vi "DevRef Data Base fg.vi"(0 "Menu":T12, 1 "Shooter Solenoid DevRef":T8={"DevStatus"={"status"=FALSE, "code"=0, "source"=""}, "Solenoid Module"=enum."Solenoid Module 1", "Forward Solenoid Channel"=enum."Invalid", "Reverse Solenoid Channel"=enum."Invalid"}, 2 "Latch Solenoid DevRef":T8={"DevStatus"={"status"=FALSE, "code"=0, "source"=""}, "Solenoid Module"=enum."Solenoid Module 1", "Forward Solenoid Channel"=enum."Invalid", "Reverse Solenoid Channel"=enum."Invalid"}, 3 "Right Up DevRef":T1={"DevStatus"={"status"=FALSE, "code"=0, "source"=""}, "DIO Channel"=enum."Invalid", "Digital Module"=enum."Digital Module 1"}, 4 "Right Down DevRef":T1={"DevStatus"={"status"=FALSE, "code"=0, "source"=""}, "DIO Channel"=enum."Invalid", "Digital Module"=enum."Digital Module 1"}, 5 "Hold Sensor DevRef":T1={"DevStatus"={"status"=FALSE, "code"=0, "source"=""}, "DIO Channel"=enum."Invalid", "Digital Module"=enum."Digital Module 1"}, 6 "2 Ball DevRef":T1={"DevStatus"={"status"=FALSE, "code"=0, "source"=""}, "DIO Channel"=enum."Invalid", "Digital Module"=enum."Digital Module 1"}, 7 "Arm Encoder DevRef":T4={"DevStatus"={"status"=FALSE, "code"=0, "source"=""}, "EncoderIndex"=enum."Invalid", "CounterIndex"=enum."Invalid", "DistancePerCount"=1.0, "Decoding Type"=enum."4x"}, 10 "DevRef to Get":T11) -> (20 "Selected Solenoid":T8={"DevStatus"={"status"=FALSE, "code"=0, "source"=""}, "Solenoid Module"=enum."Solenoid Module 1", "Forward Solenoid Channel"=enum."Invalid", "Reverse Solenoid Channel"=enum."Invalid"}, 21 "Selected Sensor":T1, 22 "Selected Encoder":T4={"DevStatus"={"status"=FALSE, "code"=0, "source"=""}, "EncoderIndex"=enum."Invalid", "CounterIndex"=enum."Invalid", "DistancePerCount"=1.0, "Decoding Type"=enum."4x"})   [LabVIEW 2013]
uses:
  <vilib>/Rock Robotics/WPI/Solenoid/WPI_SolenoidDevRef.ctl
  <vilib>/Rock Robotics/SystemInterfaces/Typedef/FPGA_TypedefSolenoidModule.ctl
  <vilib>/Rock Robotics/WPI/Solenoid/WPI_SolenoidChannel.ctl
  <vilib>/Rock Robotics/WPI/DigitalInput/WPI_DigitalInputDevRef.ctl
  <vilib>/Rock Robotics/SystemInterfaces/DIO/FPGA_DIOChannel.ctl
  <vilib>/Rock Robotics/SystemInterfaces/Typedef/FPGA_TypedefDigitalModule.ctl
  typedefs/fg_typedef.ctl
  typedefs/DevRef Type.ctl
  <vilib>/Rock Robotics/WPI/Encoder/WPI_EncoderDevRef.ctl
  <vilib>/Rock Robotics/SystemInterfaces/Encoder/FPGA_EncoderIdx.ctl
  <vilib>/Rock Robotics/SystemInterfaces/Counter/FPGA_CounterCtrSystemIndex.ctl
  <vilib>/Rock Robotics/WPI/Encoder/WPI_EncoderType.ctl
panel:
  # "A Functional Global that stores refnums for \ncommonly used devices \nso as to not need to get them repeatedly"
  # "it is only set once"
  # "Option to Select Also..."
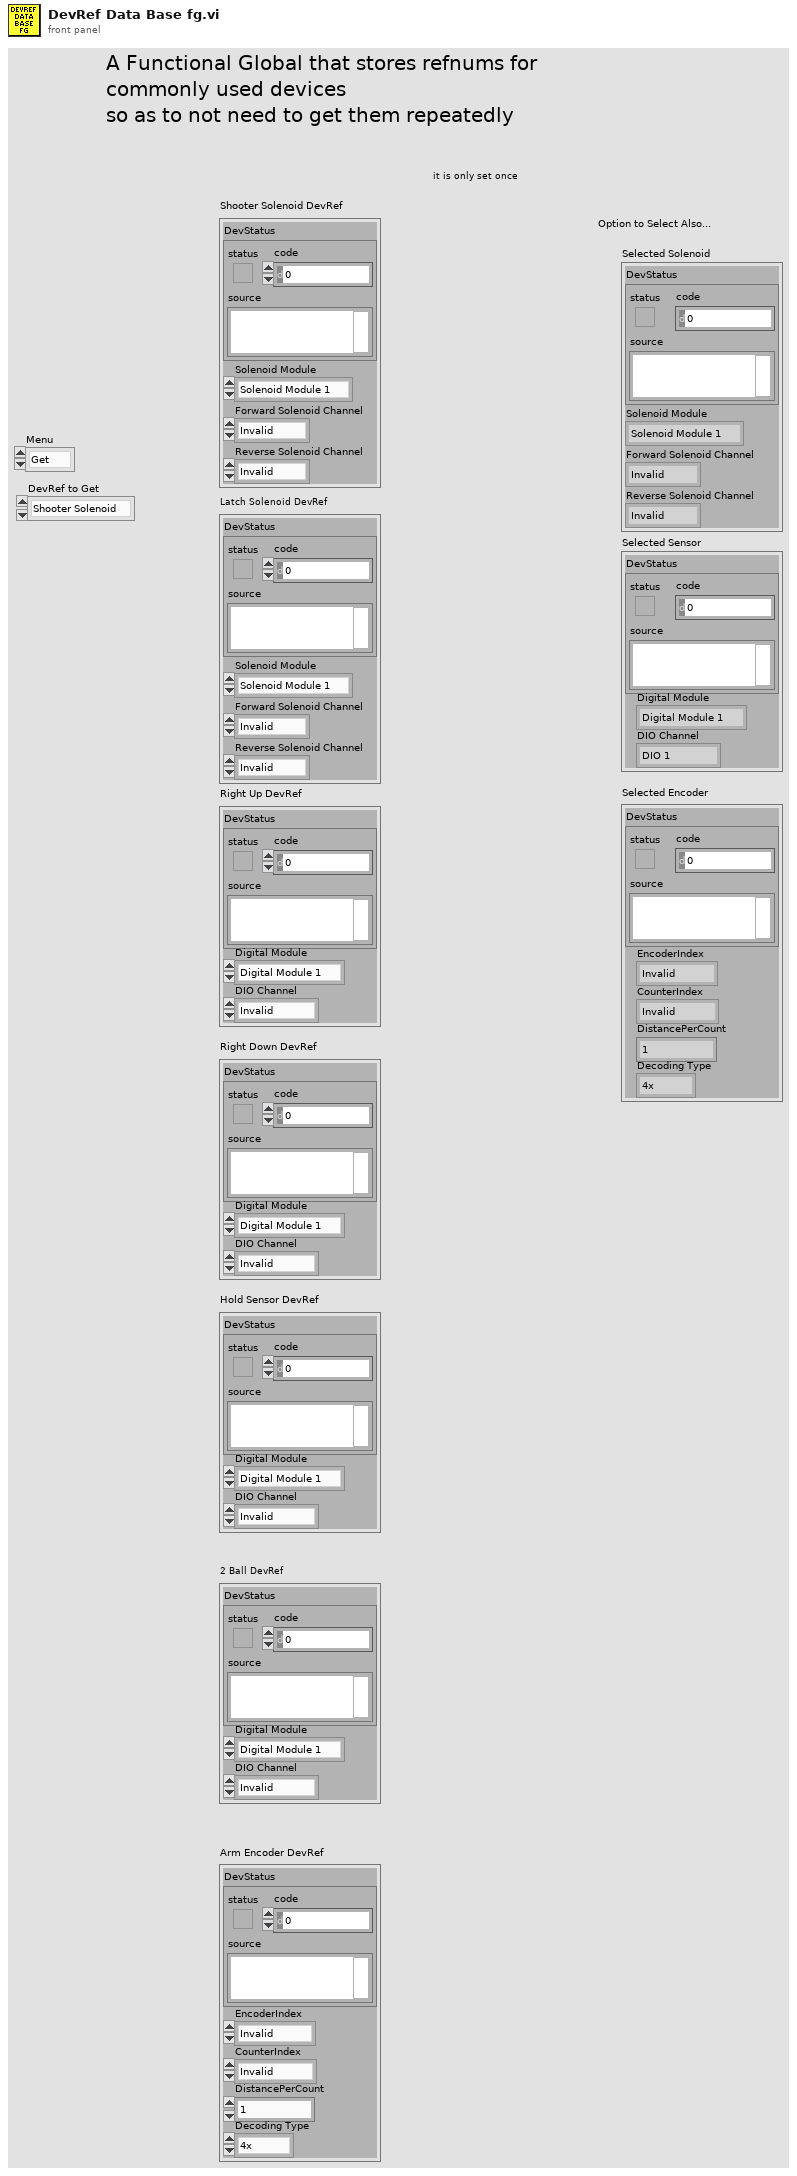
[diagram p1: front panel]
types:
  T1 = typedef "WPI_DigitalInputDevRef.ctl" = cluster{"DevStatus":errorcluster, "DIO Channel":T2, "Digital Module":T3}
  T2 = typedef "FPGA_DIOChannel.ctl" = enum8{"DIO 1", "DIO 2", "DIO 3", "DIO 4", "DIO 5", "DIO 6", "DIO 7", "DIO 8", "DIO 9", "DIO 10", "DIO 11", "DIO 12", "DIO 13", "DIO 14", "Invalid"}
  T3 = typedef "FPGA_TypedefDigitalModule.ctl" = enum16{"Digital Module 1", "Digital Module 2"}
  T4 = typedef "WPI_EncoderDevRef.ctl" = cluster{"DevStatus":errorcluster, "EncoderIndex":T5, "CounterIndex":T6, "DistancePerCount":dbl, "Decoding Type":T7}
  T5 = typedef "FPGA_EncoderIdx.ctl" = enum8{"Enc 0", "Enc 1", "Enc 2", "Enc 3", "Invalid"}
  T6 = typedef "FPGA_CounterCtrSystemIndex.ctl" = enum8{"Ctr 0", "Ctr 1", "Ctr 2", "Ctr 3", "Ctr 4", "Ctr 5", "Ctr 6", "Ctr 7", "Invalid"}
  T7 = typedef "WPI_EncoderType.ctl" = enum16{"1x", "2x", "4x"}
  T8 = typedef "WPI_SolenoidDevRef.ctl" = cluster{"DevStatus":errorcluster, "Solenoid Module":T9, "Forward Solenoid Channel":T10, "Reverse Solenoid Channel":T10}
  T9 = typedef "FPGA_TypedefSolenoidModule.ctl" = enum16{"Solenoid Module 1", "Solenoid Module 2"}
  T10 = typedef "WPI_SolenoidChannel.ctl" = enum8{"Solenoid 1", "Solenoid 2", "Solenoid 3", "Solenoid 4", "Solenoid 5", "Solenoid 6", "Solenoid 7", "Solenoid 8", "Invalid"}
  T11 = typedef "DevRef Type.ctl" = enum16{"Shooter Solenoid", "Latch Solenoid", "Right Up Sensor", "Right Down Sensor", "Hold Sensor", "2 Ball Switch", "Arm Encoder"}
  T12 = typedef "fg_typedef.ctl" = enum16{"Get", "Set"}
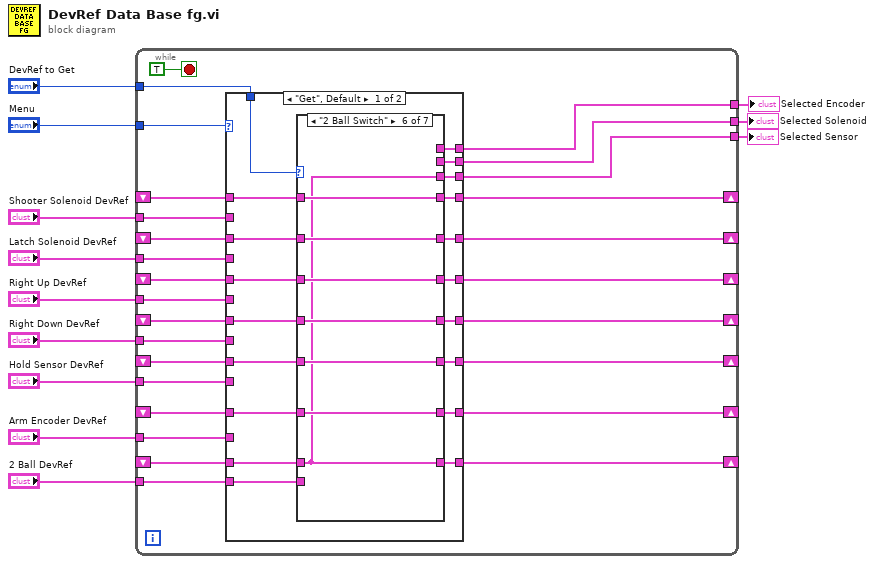
[diagram p0: block diagram]
diagram:
  n1 = while {
    shift-right: [w33] -> _
    shift-left: _ -> [w38]
    shift-right: [w32] -> _
    shift-left: _ -> [w37]
    shift-right: [w31] -> _
    shift-left: _ -> [w35]
    shift-right: [w30] -> _
    shift-left: _ -> [w34]
    tunnel: "Menu" -> [w36]
    tunnel: "Shooter Solenoid DevRef" -> [w29]
    tunnel: "Latch Solenoid DevRef" -> [w28]
    tunnel: "Right Up DevRef" -> [w27]
    tunnel: "Right Down DevRef" -> [w26]
    shift-right: [w23] -> _
    shift-left: _ -> [w24]
    tunnel: "Hold Sensor DevRef" -> [w25]
    tunnel: "DevRef to Get" -> [w22]
    tunnel: [w21] -> w5
    tunnel: [w20] -> w4
    tunnel: "Arm Encoder DevRef" -> [w19]
    shift-right: [w17] -> _
    shift-left: _ -> [w18]
    tunnel: [w16] -> w2
    tunnel: "2 Ball DevRef" -> [w15]
    shift-right: [w14] -> _
    shift-left: _ -> [w13]
    stop <- TRUE stop-if-true
    n2 = case shown="\"Get\", Default" w36 {
      tunnel: w38 -> [w57 _]
      tunnel: w37 -> [w56 _]
      tunnel: w35 -> [w55 _]
      tunnel: w34 -> [w54 _]
      tunnel: [w46 w114] -> w33
      tunnel: [w47 w113] -> w32
      tunnel: [w48 w112] -> w31
      tunnel: [w49 w111] -> w30
      tunnel: w29 -> [_ w114]
      tunnel: w28 -> [_ w113]
      tunnel: w27 -> [_ w112]
      tunnel: w26 -> [_ w111]
      tunnel: w25 -> [_ w110]
      tunnel: w24 -> [w53 _]
      tunnel: [w50 w110] -> w23
      tunnel: w22 -> [w58 _]
      tunnel: [w52 _] -> w21
      tunnel: [w51 _] -> w20
      tunnel: w19 -> [_ w109]
      tunnel: w18 -> [w45 _]
      tunnel: [w44 w109] -> w17
      tunnel: [w43 _] -> w16
      tunnel: w15 -> [w40 w108]
      tunnel: [w42 w108] -> w14
      tunnel: w13 -> [w41 _]
      frame "Get", Default {
        n3 = case shown="\"2 Ball Switch\"" w58 {
          tunnel: w57 -> [w61 w72 w79 w86 w93 w95 w107]
          tunnel: w56 -> [w62 w71 w78 w85 w92 w96 w106]
          tunnel: w55 -> [w63 w70 w77 w84 w91 w97 w105]
          tunnel: w54 -> [w64 w69 w76 w83 w90 w98 w104]
          tunnel: w53 -> [w65 w68 w75 w82 w89 w99 w103]
          tunnel: [w61 w71 _ _ _ _ _] -> w52
          tunnel: [_ _ w77 w83 w89 w94 _] -> w51
          tunnel: [w65 w68 w75 w82 w89 w99 w103] -> w50
          tunnel: [w64 w69 w76 w83 w90 w98 w104] -> w49
          tunnel: [w63 w70 w77 w84 w91 w97 w105] -> w48
          tunnel: [w62 w71 w78 w85 w92 w96 w106] -> w47
          tunnel: [w61 w72 w79 w86 w93 w95 w107] -> w46
          tunnel: w45 -> [w60 w67 w74 w81 w88 w100 w102]
          tunnel: [w60 w67 w74 w81 w88 w100 w102] -> w44
          tunnel: [_ _ _ _ _ _ w102] -> w43
          tunnel: [w59 w66 w73 w80 w87 w94 w101] -> w42
          tunnel: w41 -> [w59 w66 w73 w80 w87 w94 w101]
          tunnel: w40 -> [_ _ _ _ _ _ _]
          frame "Shooter Solenoid", Default {
          }
          frame "Latch Solenoid" {
          }
          frame "Right Up Sensor" {
          }
          frame "Right Down Sensor" {
          }
          frame "Hold Sensor" {
          }
          frame "2 Ball Switch" {
          }
          frame "Arm Encoder" {
          }
        }
      }
      frame "Set" {
      }
    }
  }
  "Selected Solenoid" <- w5
  "Selected Sensor" <- w4
  "Selected Encoder" <- w2
